vi "Get Name.vi"(8 "error in (no error)":errorcluster, 11 "Event in":refnum<class "Event.lvclass">) -> (0 "error out":errorcluster, 2 "Name out":string, 3 "Event out":refnum<class "Event.lvclass">)   [LabVIEW 2013, in "MDSplus.lvlib" / "Event.lvclass"]
doc: "Return the name associated with this event instance."
uses:
  <vilib>/MDSplus/Classes/Event_Class/Event.lvclass
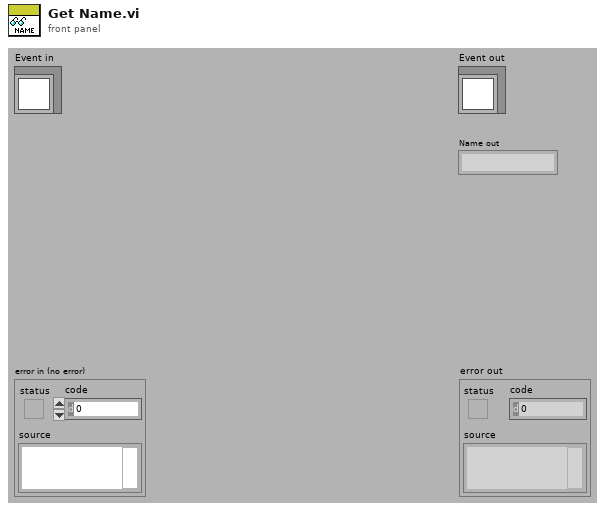
[diagram p1: front panel]
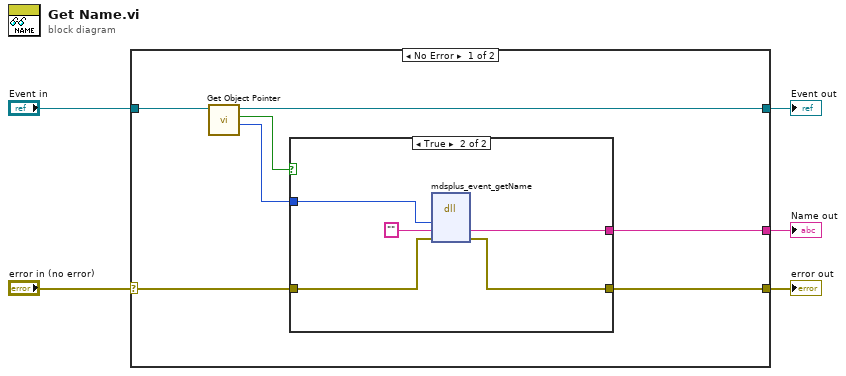
[diagram p0: block diagram]
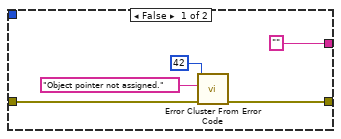
[diagram p2: hidden frame]
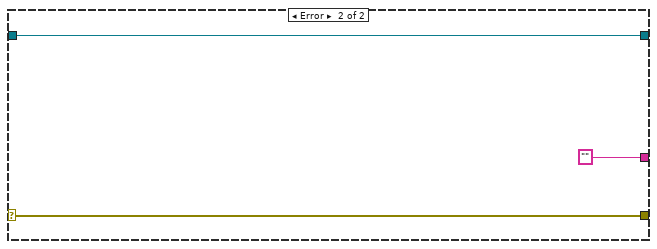
[diagram p3: hidden frame]
diagram:
  n1 = case shown="No Error" "error in (no error)" {
    selector: "error in (no error)" -> [w7 w25]
    tunnel: [w6 w25] -> w4
    tunnel: [w10 w24] -> w2
    tunnel: "Event in" -> [w11 w24]
    tunnel: [w12 "" ("size")] -> w1
    frame No Error {
      n2 = call-dynamic "Get Object Pointer.vi"("Event in"=w11) -> ("Object Pointer"=w8:i64, "Assigned object pointer?"=w9:bool, "Event out"=w10:refnum<class "Event.lvclass">)  [unwired: 8 in]
      n3 = case shown="True" w9 {
        tunnel: ["" ("sizeOut") w22] -> w12
        tunnel: w8 -> [_ w20]
        tunnel: w7 -> [w14 w19]
        tunnel: [w13 w18] -> w6
        frame False {
          n4 = call <vilib>:"Error Cluster From Error Code.vi"("error in (no error)"=w14, "error message (\"\")"="Object pointer not assigned." ("error message (\"\")"), "error code (0)"=42) -> ("error out"=w13:errorcluster)  [unwired: 6 in]
        }
        frame True {
          n5 = dll-call lib="MDSobjectsLVShr" fn="mdsplus_event_getName"("lvEventPtr"=w20, "lvStrHdlOut"="" ("size"), "error"=w19) -> ("lvStrHdlOut"=w22:string, "error"=w18:errorcluster)  [unwired: 5 in, 2 out]
        }
      }
    }
    frame Error {
    }
  }
  "error out" <- w4
  "Event out" <- w2
  "Name out" <- w1
